vi "Left Motor Angle Loop (SubVI).vi"   [LabVIEW 2015]
uses:
  Left Variables.vi
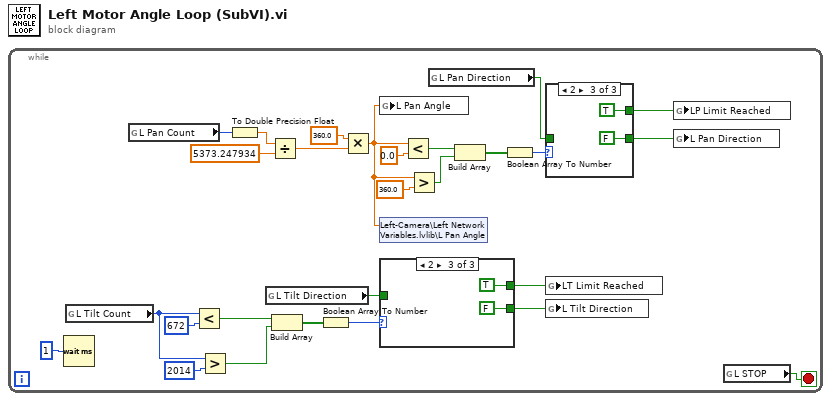
[diagram p0: block diagram]
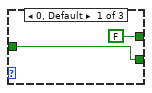
[diagram p2: hidden frame]
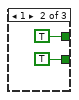
[diagram p3: hidden frame]
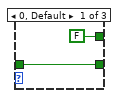
[diagram p4: hidden frame]
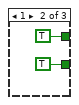
[diagram p5: hidden frame]
diagram:
  n1 = while {
    stop <- w22 stop-if-true
    n2 = Wait (ms)(milliseconds to wait=u32 1) -> ()  [unwired: 1 out]
    n3 = global read "Left Variables.vi" "L Tilt Count"() -> (w1:i32)
    n4 = global read "Left Variables.vi" "L Pan Count"() -> (w27:i32)
    n5 = Less?(x=w1, y=672 ("upper limit")) -> (x < y?=w8:bool)
    n6 = Greater?(x=w1, y=2014 ("lower limit")) -> (0:w7:bool)
    n7 = To Double Precision Float(number=w27) -> (double precision float=w24:dbl)
    n8 = global read "Left Variables.vi" "L Tilt Direction"() -> (w2:bool)
    n9 = Divide(x=w24, y=5373.247934) -> (x/y=w26:dbl)
    n10 = Build Array(w8, w7) -> (w6:bool[])
    n11 = Boolean Array To Number(Boolean array=w6) -> (number=w5:u32)
    n12 = Multiply(x=360.0, y=w26) -> (x*y=w15:dbl)
    n13 = global write "Left Variables.vi" "L Pan Angle"(w15) -> ()
    n14 = shared-variable "Left-Camera\\Left Network Variables.lvlib\\L Pan Angle"(w15) -> ()  [unwired: 1 in, 1 out]
    n15 = case shown="2" w5 {
      tunnel: [w29 TRUE FALSE] -> w4
      tunnel: w2 -> [w29 _ _]
      tunnel: [FALSE TRUE TRUE] -> w3
      frame 0, Default {
      }
      frame 1 {
      }
      frame 2 {
      }
    }
    n16 = Less?(x=w15, y=0.0) -> (x < y?=w17:bool)
    n17 = Greater?(x=w15, y=360.0) -> (0:w16:bool)
    n18 = global read "Left Variables.vi" "L Pan Direction"() -> (w14:bool)
    n19 = Build Array(w17, w16) -> (w18:bool[])
    n20 = Boolean Array To Number(Boolean array=w18) -> (number=w13:u32)
    n21 = case shown="2" w13 {
      tunnel: [w35 TRUE FALSE] -> w12
      tunnel: w14 -> [w35 _ _]
      tunnel: [FALSE TRUE TRUE] -> w11
      frame 0, Default {
      }
      frame 1 {
      }
      frame 2 {
      }
    }
    n22 = global write "Left Variables.vi" "LT Limit Reached"(w3) -> ()
    n23 = global write "Left Variables.vi" "L Tilt Direction"(w4) -> ()
    n24 = global write "Left Variables.vi" "LP Limit Reached"(w11) -> ()
    n25 = global write "Left Variables.vi" "L Pan Direction"(w12) -> ()
    n26 = global read "Left Variables.vi" "L STOP"() -> (w22:bool)
  }
